vi "1 channel N sample (temperature measurement).vi"() -> ()   [LabVIEW 2020]
panel:
  out "Array":dbl[](array[numeric])
  in  "number of samples":i32=100
  out "Waveform Graph":dynamicdata(graph)
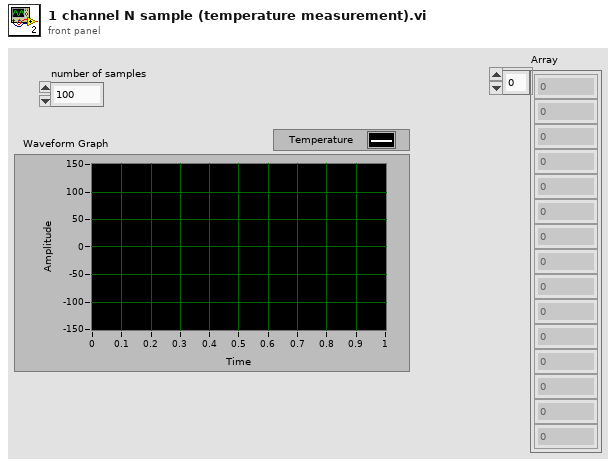
[diagram p1: front panel]
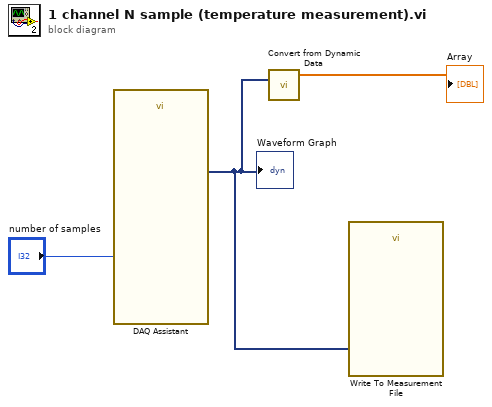
[diagram p0: block diagram]
diagram:
  n1 = call "DAQ Assistant"("number of samples"="number of samples") -> ("data"=w1:dynamicdata)  [unwired: 16 in, 2 out]
  "Waveform Graph" <- w1
  n2 = call "Convert from Dynamic Data"("Dynamic Data Type"=w1) -> ("Array"=→"Array":dbl[])  [unwired: 3 in]
  n3 = call "Write To Measurement File"("Signals"=w1) -> ()  [unwired: 16 in, 3 out]
